vi "endcvlib.vi"() -> (3 "function return":u32)   [LabVIEW 2012, in "cvlib.lvlib"]
doc: "extern \"C\" __declspec(dllexport) unsigned long __cdecl endcvlib();"
uses:
  cvlib.lvlib
  cvlib.dll
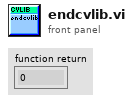
[diagram p1: front panel]
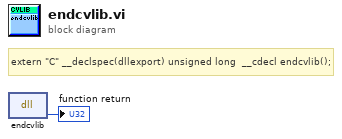
[diagram p0: block diagram]
diagram:
  # "extern \"C\" __declspec(dllexport) unsigned long \t__cdecl endcvlib();"
  n1 = dll-call lib="C:/Users/myerslab/workspace2/Libraries/ClearVolume/cpp/labview/lvcvlib/cvlib.*" fn="endcvlib"() -> (→"function return":u32)  [unwired: 3 in, 2 out]
